vi "CreateSensorInstByName.vi"(0 "Fehler (Eingang, kein Fehler)":errorcluster, 7 "DLL-Path":path, 9 "sensor":string) -> (4 "Fehler (Ausgang)":errorcluster, 6 "instanceHandle":u32, 8 "DLL-Path":path)   [LabVIEW 2015, in "MEDAQLib.lvlib"]
doc: "DWORD CreateSensorInstance (ME_SENSOR sensor);\n\nCreates an instance for the sensor which will be used in further function calls.\nAttention! Please don't forget to release the instance at the end. Otherwise\nthere will be memory and handle leaks."
uses:
  MEDAQLib.lvlib
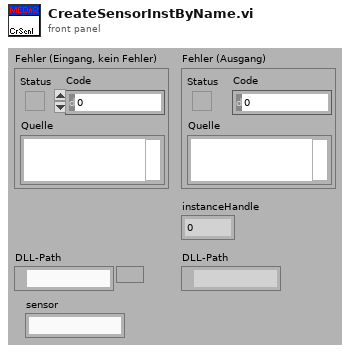
[diagram p1: front panel]
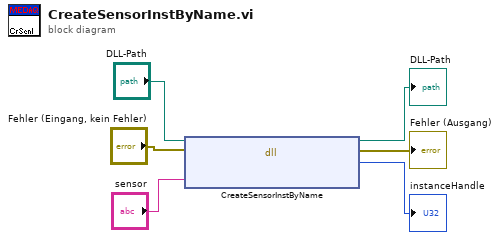
[diagram p0: block diagram]
diagram:
  n1 = dll-call lib="D:/Users/XRF/Desktop/Dante_acquire6/libs/Proximity_sensor/Release/MEDAQLib.dll" fn="CreateSensorInstByName"(path in="DLL-Path", error in="Fehler (Eingang, kein Fehler)", "sensor"="sensor") -> (path out=→"DLL-Path":path, error out=→"Fehler (Ausgang)":errorcluster, "Rückgabetyp"=→"instanceHandle":u32)  [unwired: 2 in]
